vi "SelectPath.vi"(8 "error in (no error)":errorcluster caption="error in") -> (0 "error out":errorcluster, 3 "selected path":path)   [LabVIEW 2011]
uses:
  <vilib>/Utility/sysdir.llb/System Directory Type.ctl
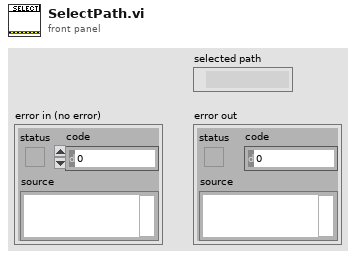
[diagram p1: front panel]
types:
  T1 = typedef "System Directory Type.ctl" = i32
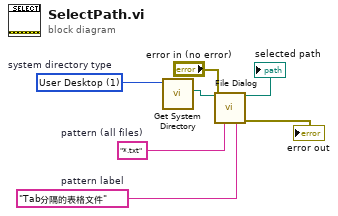
[diagram p0: block diagram]
diagram:
  w4 = "Tab分隔的表格文件"  # pattern label
  w3 = "*.txt"  # pattern (all files)
  w1 = T1 1 items=["User Home"=0, "User Desktop"=1, "User Documents"=2, "User Application Data"=3, "User Preferences"=4, "User Temporary"=5, "Public Documents"=6, "Public Application Data"=7, "Public Preferences"=8, "Public Cache"=13, "System Core Libraries"=9, "System Installed Libraries"=10, "Application Files"=11, "Boot Volume Root"=12]  # system directory type
  n1 = call <vilib>:"Get System Directory.vi"("system directory type"=w1) -> ("system directory"=w2:path)  [unwired: 10 in]
  n2 = call "File Dialog"("start path"=w2, "error in"="error in (no error)", "pattern (all files)"=w3, "pattern label"=w4) -> ("selected path"=→"selected path":path, "error out"=→"error out":errorcluster)  [unwired: 8 in, 2 out]
